vi "2.vi"(9 "Range end":dbl=10.0, 10 "Step in":dbl=1.0, 11 "Range start in":dbl) -> (1 "Boolean":bool, 2 "Range start out":dbl, 3 "Numeric":dbl, 4 "Step out":dbl)   [LabVIEW 2020]
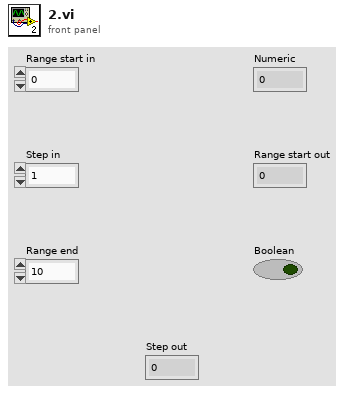
[diagram p1: front panel]
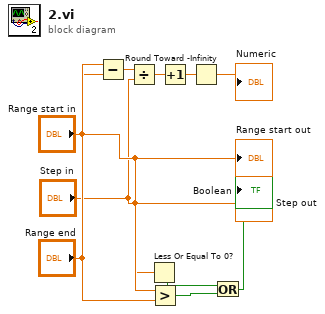
[diagram p0: block diagram]
diagram:
  n1 = Subtract(x="Range end", y="Range start in") -> (x-y=w1:dbl)
  n2 = Divide(x=w1, y="Step in") -> (x/y=w2:dbl)
  n3 = Less Or Equal To 0?(x="Step in") -> (x <= 0?=w6:bool)
  n4 = Greater?(x="Range start in", y="Range end") -> (0:w7:bool)
  n5 = Increment(x=w2) -> (x+1=w3:dbl)
  n6 = Round Toward -Infinity(1:w3) -> (0:→"Numeric":dbl)
  n7 = Or(x=w6, y=w7) -> (x .or. y?=→"Boolean":bool)
  "Range start out" <- "Range start in"
  "Step out" <- "Step in"
